vi "Rig - Create New.vi"(8 "Error IN":errorcluster, 11 "Existing Rig Config Names":string[](array[string])) -> (0 "Error OUT":errorcluster, 1 "Cancel OUT":bool, 3 "Enter New Rig Config File Name OUT":string)   [LabVIEW 2018]
panel:
  in  "Enter New Rig Config File Name":string
  in  "Cancel":bool
  in  "Next":bool
  # "New Rig File Name"
  # ".dat"
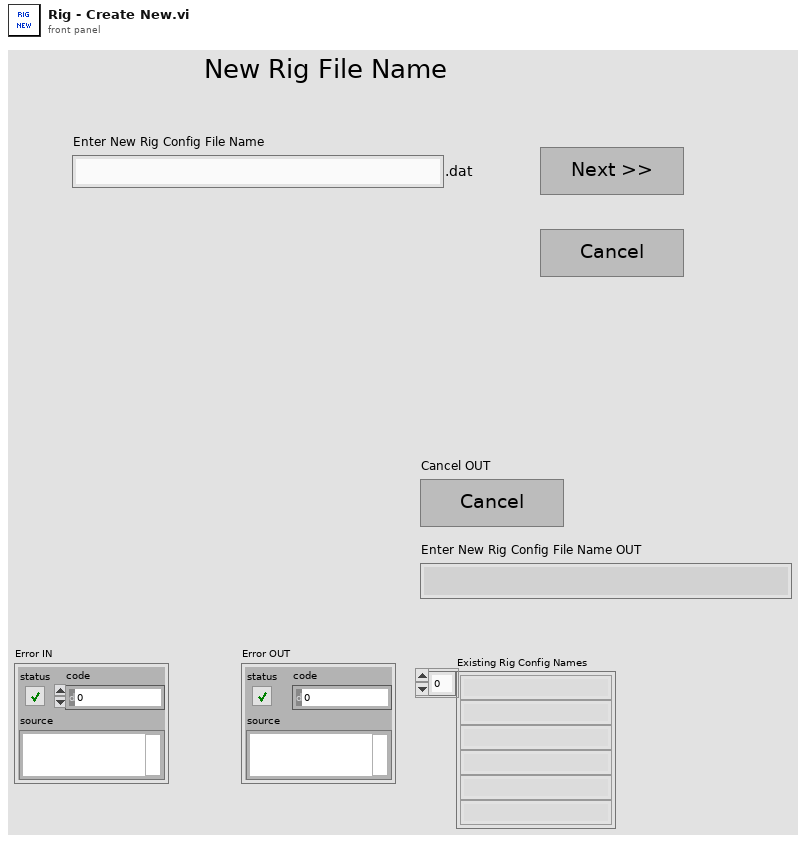
[diagram p1: front panel]
types:
  T1 = enum8{"Enabled", "Disabled", "Disabled and Grayed Out"}
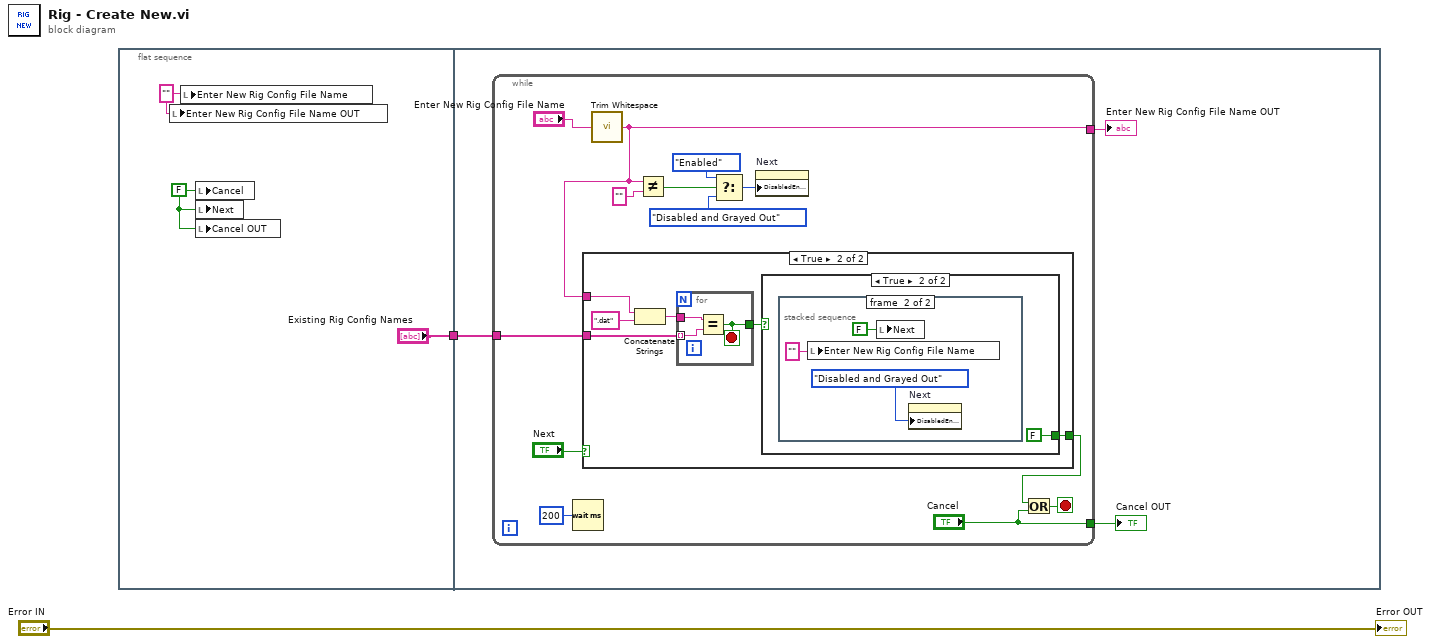
[diagram p0: block diagram]
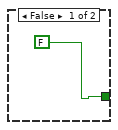
[diagram p2: hidden frame]
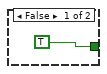
[diagram p3: hidden frame]
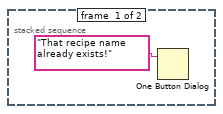
[diagram p4: hidden frame]
diagram:
  n1 = flat-sequence {
    tunnel: ["Existing Rig Config Names"] -> w1
    tunnel: w1 -> [w7]
    frame #0 {
      w4 = FALSE ("Cancel")
      w5 = "" ("Enter New Recipe File Name")
      n2 = local write "Enter New Rig Config File Name OUT"(w5) -> ()
      n3 = local write "Enter New Rig Config File Name"(w5) -> ()
      n4 = local write "Cancel"(w4) -> ()
      n5 = local write "Next"(w4) -> ()
      n6 = local write "Cancel OUT"(w4) -> ()
    }
    frame #1 {
      n7 = while {
        tunnel: [w9] -> w6
        tunnel: ["Cancel"] -> w8
        tunnel: w7 -> [w12]
        stop <- w21 stop-if-true
        n8 = Wait (ms)(milliseconds to wait=u32 200) -> ()  [unwired: 1 out]
        n9 = call <vilib>:"Trim Whitespace.vi"("string"="Enter New Rig Config File Name") -> ("trimmed string"=w9:string)  [unwired: 1 in]
        n10 = case shown="True" "Next" {
          tunnel: w9 -> [_ w25]
          tunnel: w12 -> [_ w28]
          tunnel: [FALSE w26] -> w11
          frame False {
          }
          frame True {
            n11 = Concatenate Strings(w25, ".dat" ("string")) -> (w24:string)
            n12 = for {
              tunnel: w28 -> [w36] mode=indexing
              tunnel: w24 -> [w37]
              tunnel: [w35] -> w27
              stop <- w35 stop-if-true
              n13 = Equal?(x=w37, y=w36) -> (x = y?=w35:bool)
            }
            n14 = case shown="True" w27 {
              tunnel: [TRUE FALSE] -> w26
              frame False {
              }
              frame True {
                n15 = stacked-sequence {
                  frame #0 {
                    n16 = One Button Dialog(message="That recipe name already exists!") -> ()  [unwired: 1 in, 1 out]
                  }
                  frame #1 {
                    n17 = local write "Enter New Rig Config File Name"("" ("Enter New Recipe File Name")) -> ()
                    n18 = local write "Next"(FALSE ("Next")) -> ()
                    n19 = property on="Next" class="Bool (strict)"("DisabledEnum"=T1."Disabled and Grayed Out" ("Disabled")) -> ()  [unwired: 2 in, 2 out]
                  }
                }
              }
            }
          }
        }
        n20 = Not Equal?(x=w9, y="") -> (x != y?=w18:bool)
        n21 = Select(t=T1."Enabled" ("Disabled"), s=w18, f=T1."Disabled and Grayed Out" ("Disabled")) -> (s? t:f=w15:T1)
        n22 = property on="Next" class="Bool (strict)"("DisabledEnum"=w15) -> ()  [unwired: 2 in, 2 out]
        n23 = Or(x=w11, y="Cancel") -> (x .or. y?=w21:bool)
      }
      "Enter New Rig Config File Name OUT" <- w6
      "Cancel OUT" <- w8
    }
  }
  "Error OUT" <- "Error IN"
